vi "Write tag select.vi"(8 "error in":errorcluster, 10 "tag select":T1[](array[typedef]), 11 "tag select module configuration in":refnum<class "Table Test configuration.lvclass">) -> (0 "error out":errorcluster, 3 "tag select module configuration out":refnum<class "Table Test configuration.lvclass">)   [LabVIEW 2013, in "Table Test configuration.lvclass"]
uses:
  Table Test configuration.lvclass
  tag select configuration.ctl
  <vilib>/NI/Tag Bus Module Framework/channel/TBM channel.lvclass
  <vilib>/NI/Tag Bus/tag/Data Type.ctl
  Table Test configuration.lvclass/Table Test configuration.ctl
  <vilib>/NI/Tag Bus/tag/tag descriptor.lvclass
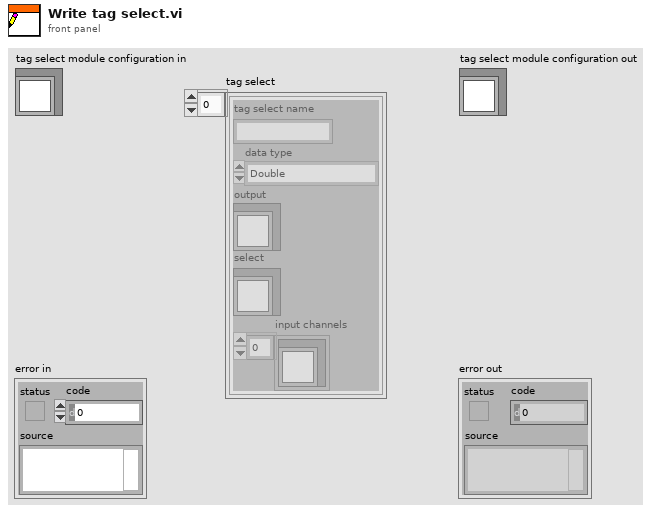
[diagram p1: front panel]
types:
  T1 = typedef "Table Test configuration.lvclass/tag select configuration.ctl" = cluster{"tag select name":string, "data type":T2, "output":refnum<class "TBM channel.lvclass">, "select":refnum<class "TBM channel.lvclass">, "input channels":refnum<class "TBM channel.lvclass">[]}
  T2 = typedef "tag bus.lvlib/tag descriptor.lvclass/Data Type.ctl" = enum16{"Double", "Single", "I64", "I32", "I16", "I8", "U64", "U32", "U16", "U8", "Boolean", "String", "Array of Double", "Array of Single", "Array of I64", "Array of I32", "Array of I16", "Array of I8", "Array of U64", "Array of U32", "Array of U16", "Array of U8", "Array of Boolean", "Array of String"}
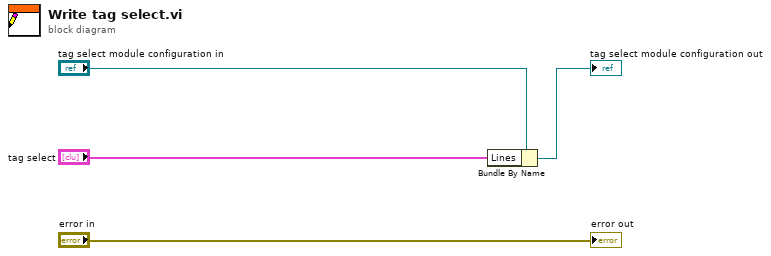
[diagram p0: block diagram]
diagram:
  n1 = Bundle By Name(cluster="tag select module configuration in", "Lines"="tag select") -> (→"tag select module configuration out":refnum<class "Table Test configuration.lvclass">)
  "error out" <- "error in"
